vi "Command line.vi"() -> ()   [LabVIEW 2015]
panel:
  out "error out":errorcluster
  out "return code":i32
  out "standard error":string
  out "standard output":string
  in  "run minimized? (F)":bool=TRUE
  in  "error in (no error)":errorcluster
  in  "working directory":path=path "c:/3"
  in  "standard input":string
  in  "expected output size  (4096)":u32=4096
  in  "wait until completion? (T)":bool=TRUE
  in  "command line":string="cmd.exe /c client.py -a 192.168.1.3 -t7 -i ab.gif"
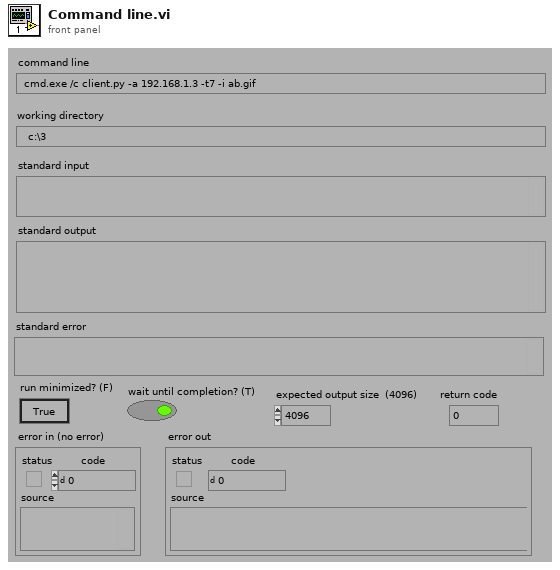
[diagram p1: front panel]
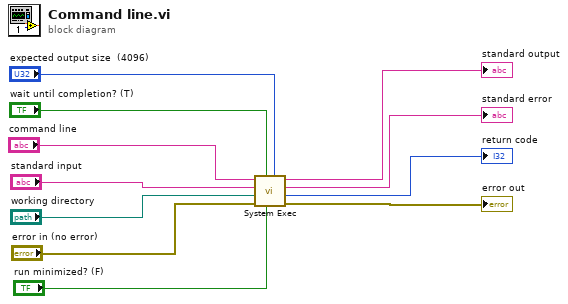
[diagram p0: block diagram]
diagram:
  n1 = call <vilib>:"System Exec.vi"("expected output size  (4096)"="expected output size  (4096)", "run minimized? (F)"="run minimized? (F)", "wait until completion? (T)"="wait until completion? (T)", "error in (no error)"="error in (no error)", "working directory"="working directory", "standard input"="standard input", "command line"="command line") -> ("error out"=→"error out":errorcluster, "return code"=→"return code":i32, "standard error"=→"standard error":string, "standard output"=→"standard output":string)  [unwired: 1 in]
